vi "Teleop Cmd Send.vi"(0 "rt fifo":refnum<k33>, 1 "Cluster":T1, 3 "error in (no error)":errorcluster, 4 "Epsilon":dbl) -> (10 "error out":errorcluster)   [LabVIEW 2013]
uses:
  dashboard/TeleopCmd.ctl
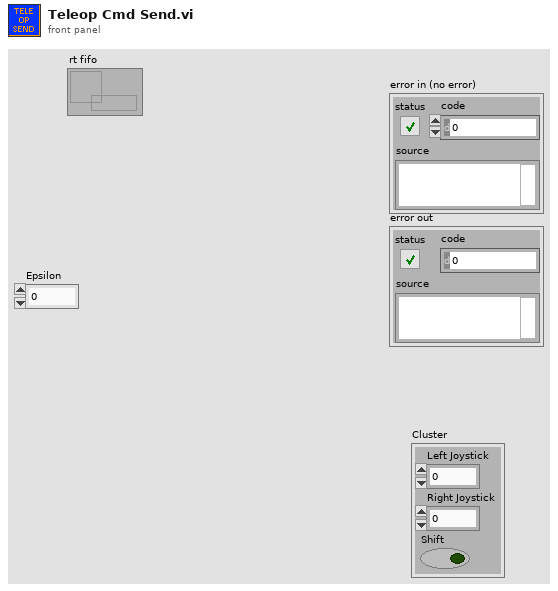
[diagram p1: front panel]
types:
  T1 = typedef "TeleopCmd.ctl" = cluster{"Left Joystick":dbl, "Right Joystick":dbl, "Shift":bool}
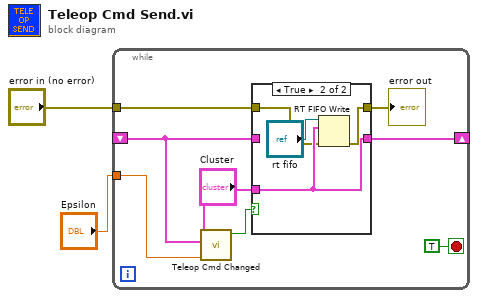
[diagram p0: block diagram]
diagram:
  n1 = while "Prev Right\nPrev Right Value" {
    tunnel: "error in (no error)" -> [w7]
    tunnel: "Epsilon" -> [w5]
    shift-right: [w4] -> _
    shift-left: _ -> [w3]
    stop <- TRUE stop-if-true
    n2 = call "Teleop Cmd Changed.vi"("Epsilon"=w5, "New Teleop Values"=w3, "Prev Teleop Values"="Cluster") -> ("Boolean"=w9:bool)  [unwired: 8 in]
    n3 = case shown="True" w9 {
      tunnel: [w12 w16] -> w8
      tunnel: w7 -> [w12 w13]
      tunnel: "Cluster" -> [_ w14]
      tunnel: [w11 w14] -> w4
      tunnel: w3 -> [w11 _]
      frame False {
      }
      frame True {
        n4 = RT FIFO Write(0:"rt fifo", 1:w14, 3:w13) -> (11:w16:errorcluster)  [unwired: 2 in, 3 out]
      }
    }
    "error out" <- w8
  }
